vi "waveformGenerator.vi"() -> ()   [LabVIEW 2020]
panel:
  out "Waveform Graph 8":dbl[](graph)
  out "Sawtooth":string
  out "Waveform Graph 7":dbl[](graph)
  out "Square":string
  out "Waveform Graph 6":dbl[](graph)
  out "Camel Sine":string
  out "Waveform Graph 5":dbl[](graph)
  out "Alternating Sine":string
  out "Waveform Graph 4":dbl[](graph)
  out "Pulse Sine":string
  out "Waveform Graph 3":dbl[](graph)
  out "Abs Sine":string
  out "Waveform Graph 2":dbl[](graph)
  out "Half Sine":string
  out "Waveform Graph":dbl[](graph)
  out "Sine":string
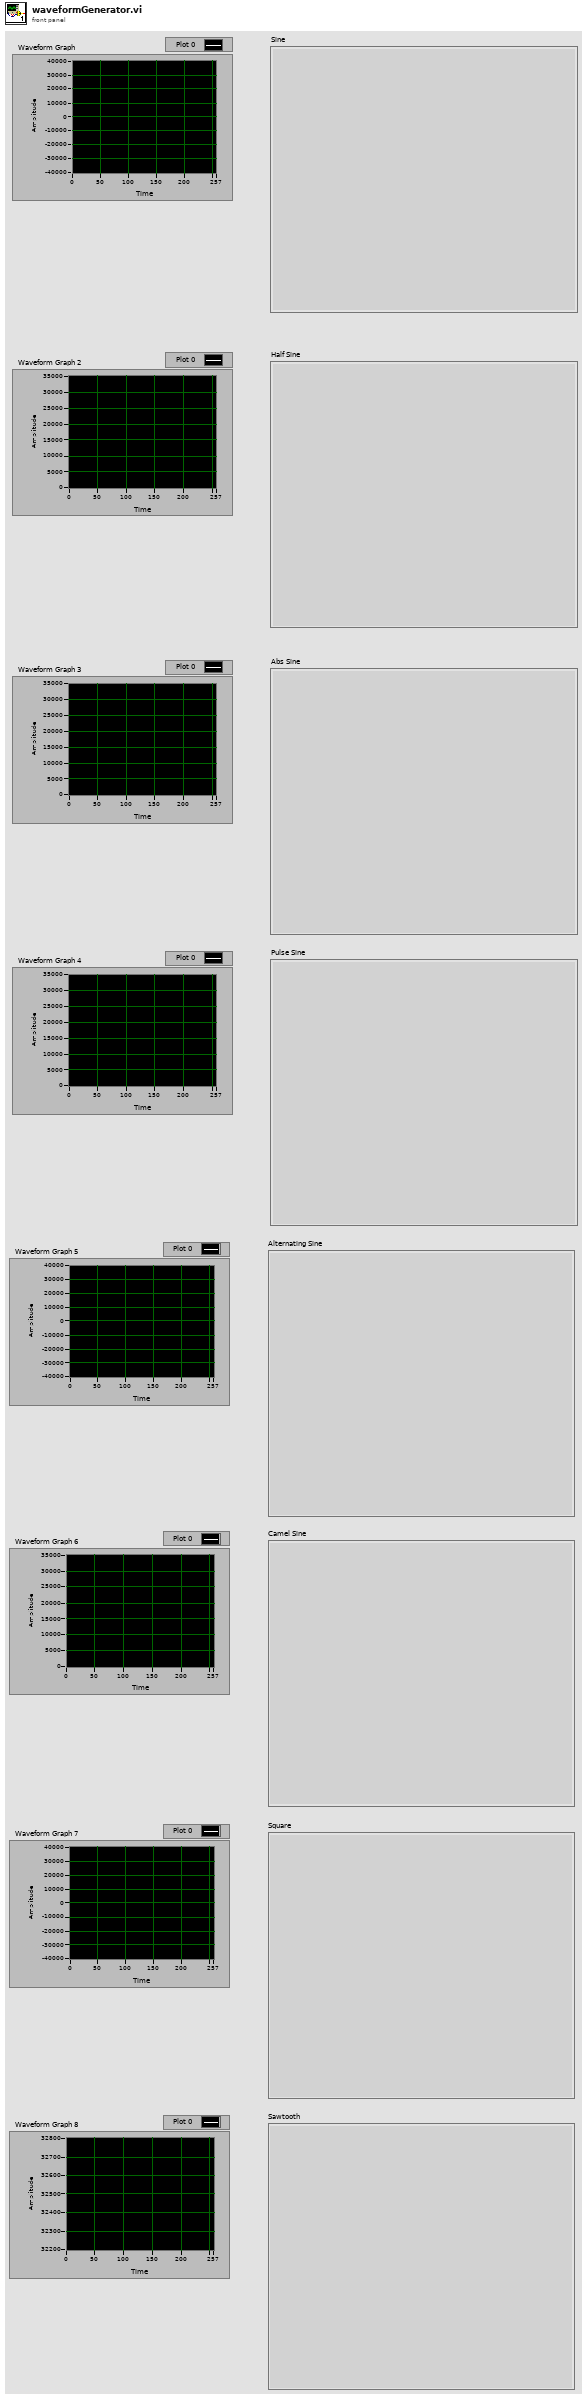
[diagram p1: front panel]
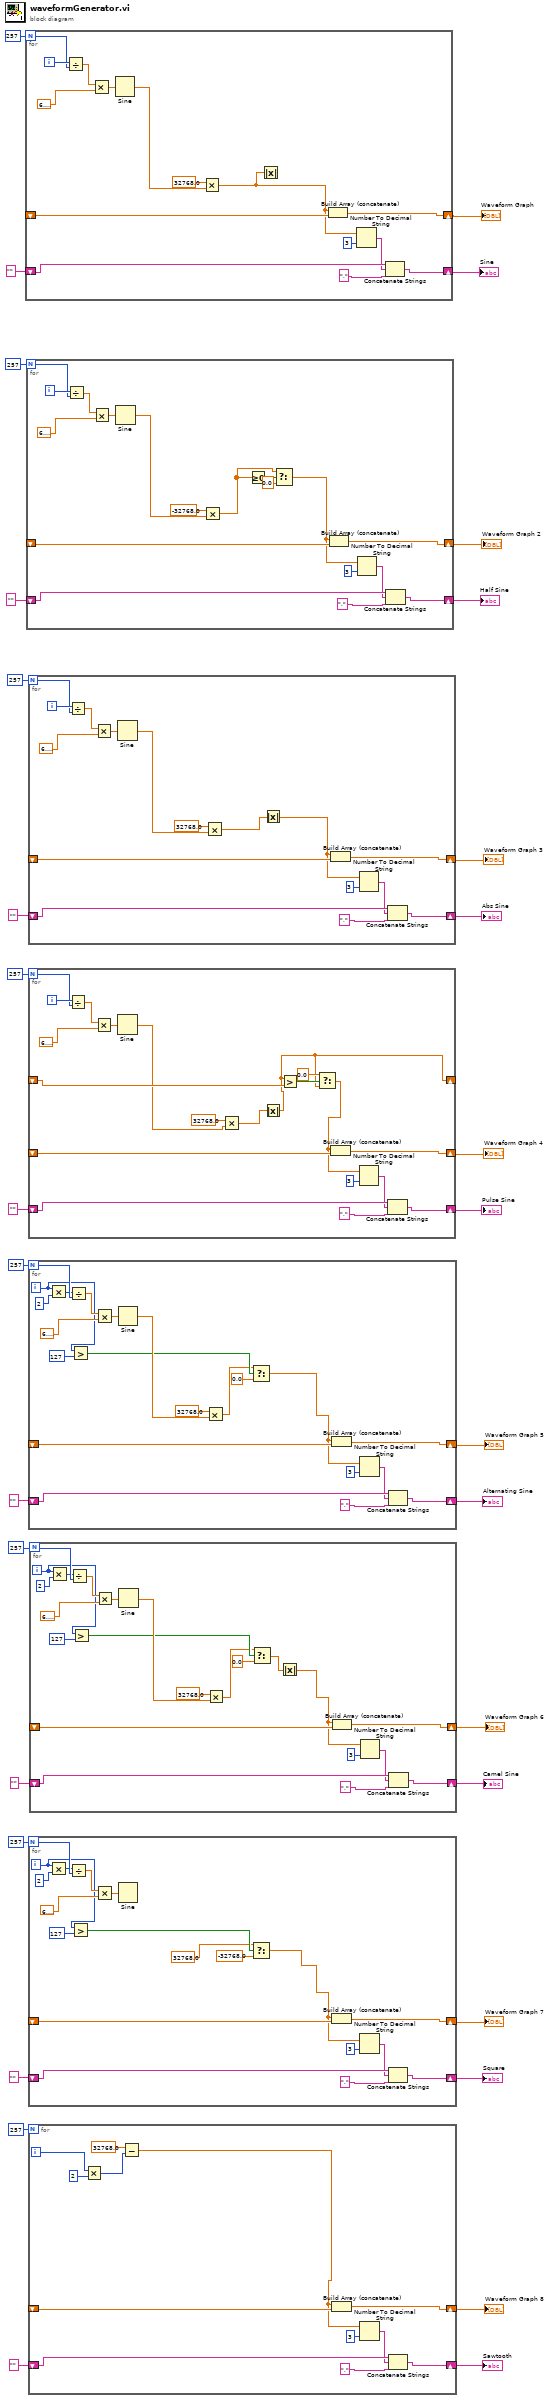
[diagram p0: block diagram]
diagram:
  n1 = for {
    N: 257 -> [w46]
    shift-right: [w39] -> w31
    shift-left: "" ("String") -> [w40]
    shift-right: [w41] -> w29
    shift-left: _ -> [w42]
    i -> [w47]
    n2 = Divide(x=w47, y=w46) -> (x/y=w44:dbl)
    n3 = Multiply(x=w44, y=6.283185307179586) -> (x*y=w43:dbl)
    n4 = Sine(x=w43) -> (sin(x)=w37:dbl)
    n5 = Multiply(x=32768.0, y=w37) -> (x*y=w35:dbl)
    n6 = Absolute Value(x=w35) -> ()  [unwired: 1 out]
    n7 = Build Array (concatenate)(w35, w42) -> (w41:dbl[])
    n8 = Number To Decimal String(number=w35, width (-)=i16 3) -> (decimal integer string=w34:string)
    n9 = Concatenate Strings(w40, w34, "," ("string")) -> (w39:string)
  }
  "Sine" <- w31
  "Waveform Graph" <- w29
  n10 = for {
    N: 257 -> [w64]
    shift-right: [w57] -> w27
    shift-left: "" ("String") -> [w58]
    shift-right: [w59] -> w25
    shift-left: _ -> [w60]
    i -> [w65]
    n11 = Divide(x=w65, y=w64) -> (x/y=w62:dbl)
    n12 = Multiply(x=w62, y=6.283185307179586) -> (x*y=w61:dbl)
    n13 = Sine(x=w61) -> (sin(x)=w55:dbl)
    n14 = Multiply(x=-32768.0, y=w55) -> (x*y=w50:dbl)
    n15 = Greater Or Equal To 0?(x=w50) -> (x >= 0?=w51:bool)
    n16 = Select(t=w50, s=w51, f=0.0) -> (s? t:f=w48:dbl)
    n17 = Build Array (concatenate)(w48, w60) -> (w59:dbl[])
    n18 = Number To Decimal String(number=w48, width (-)=i16 3) -> (decimal integer string=w53:string)
    n19 = Concatenate Strings(w58, w53, "," ("string")) -> (w57:string)
  }
  "Half Sine" <- w27
  "Waveform Graph 2" <- w25
  n20 = for {
    N: 257 -> [w80]
    shift-right: [w73] -> w23
    shift-left: "" ("String") -> [w74]
    shift-right: [w75] -> w21
    shift-left: _ -> [w76]
    i -> [w81]
    n21 = Divide(x=w81, y=w80) -> (x/y=w78:dbl)
    n22 = Multiply(x=w78, y=6.283185307179586) -> (x*y=w77:dbl)
    n23 = Sine(x=w77) -> (sin(x)=w71:dbl)
    n24 = Multiply(x=32768.0, y=w71) -> (x*y=w69:dbl)
    n25 = Absolute Value(x=w69) -> (abs(x)=w66:dbl)
    n26 = Build Array (concatenate)(w66, w76) -> (w75:dbl[])
    n27 = Number To Decimal String(number=w66, width (-)=i16 3) -> (decimal integer string=w68:string)
    n28 = Concatenate Strings(w74, w68, "," ("string")) -> (w73:string)
  }
  "Abs Sine" <- w23
  "Waveform Graph 3" <- w21
  n29 = for {
    N: 257 -> [w100]
    shift-right: [w93] -> w19
    shift-left: "" ("String") -> [w94]
    shift-right: [w95] -> w17
    shift-left: _ -> [w96]
    shift-right: [w82] -> _
    shift-left: _ -> [w87]
    i -> [w101]
    n30 = Divide(x=w101, y=w100) -> (x/y=w98:dbl)
    n31 = Multiply(x=w98, y=6.283185307179586) -> (x*y=w97:dbl)
    n32 = Sine(x=w97) -> (sin(x)=w83:dbl)
    n33 = Multiply(x=32768.0, y=w83) -> (x*y=w90:dbl)
    n34 = Absolute Value(x=w90) -> (abs(x)=w82:dbl)
    n35 = Greater?(x=w82, y=w87) -> (0:w86:bool)
    n36 = Select(t=0.0, s=w86, f=w82) -> (s? t:f=w84:dbl)
    n37 = Build Array (concatenate)(w84, w96) -> (w95:dbl[])
    n38 = Number To Decimal String(number=w84, width (-)=i16 3) -> (decimal integer string=w89:string)
    n39 = Concatenate Strings(w94, w89, "," ("string")) -> (w93:string)
  }
  "Pulse Sine" <- w19
  "Waveform Graph 4" <- w17
  n40 = for {
    N: 257 -> [w122]
    shift-right: [w115] -> w15
    shift-left: "" ("String") -> [w116]
    shift-right: [w117] -> w13
    shift-left: _ -> [w118]
    i -> [w107]
    n41 = Multiply(x=w107, y=2) -> (x*y=w109:i32)
    n42 = Divide(x=w109, y=w122) -> (x/y=w120:dbl)
    n43 = Greater?(x=w107, y=127) -> (0:w105:bool)
    n44 = Multiply(x=w120, y=6.283185307179586) -> (x*y=w119:dbl)
    n45 = Sine(x=w119) -> (sin(x)=w113:dbl)
    n46 = Multiply(x=32768.0, y=w113) -> (x*y=w104:dbl)
    n47 = Select(t=w104, s=w105, f=0.0) -> (s? t:f=w103:dbl)
    n48 = Build Array (concatenate)(w103, w118) -> (w117:dbl[])
    n49 = Number To Decimal String(number=w103, width (-)=i16 3) -> (decimal integer string=w111:string)
    n50 = Concatenate Strings(w116, w111, "," ("string")) -> (w115:string)
  }
  "Alternating Sine" <- w15
  "Waveform Graph 5" <- w13
  n51 = for {
    N: 257 -> [w141]
    shift-right: [w134] -> w7
    shift-left: "" ("String") -> [w135]
    shift-right: [w136] -> w5
    shift-left: _ -> [w137]
    i -> [w128]
    n52 = Multiply(x=w128, y=2) -> (x*y=w130:i32)
    n53 = Divide(x=w130, y=w141) -> (x/y=w139:dbl)
    n54 = Greater?(x=w128, y=127) -> (0:w126:bool)
    n55 = Multiply(x=w139, y=6.283185307179586) -> (x*y=w138:dbl)
    n56 = Sine(x=w138) -> ()  [unwired: 1 out]
    n57 = Select(t=32768.0 ("x"), s=w126, f=-32768.0) -> (s? t:f=w123:dbl)
    n58 = Build Array (concatenate)(w123, w137) -> (w136:dbl[])
    n59 = Number To Decimal String(number=w123, width (-)=i16 3) -> (decimal integer string=w132:string)
    n60 = Concatenate Strings(w135, w132, "," ("string")) -> (w134:string)
  }
  "Square" <- w7
  "Waveform Graph 7" <- w5
  n61 = for {
    N: 257 -> [_]
    shift-right: [w150] -> w3
    shift-left: "" ("String") -> [w151]
    shift-right: [w152] -> w1
    shift-left: _ -> [w153]
    i -> [w145]
    n62 = Multiply(x=w145, y=2) -> (x*y=w144:i32)
    n63 = Subtract(x=32768.0, y=w144) -> (x-y=w142:dbl)
    n64 = Build Array (concatenate)(w142, w153) -> (w152:dbl[])
    n65 = Number To Decimal String(number=w142, width (-)=i16 3) -> (decimal integer string=w148:string)
    n66 = Concatenate Strings(w151, w148, "," ("string")) -> (w150:string)
  }
  "Sawtooth" <- w3
  "Waveform Graph 8" <- w1
  n67 = for {
    N: 257 -> [w175]
    shift-right: [w168] -> w11
    shift-left: "" ("String") -> [w169]
    shift-right: [w170] -> w9
    shift-left: _ -> [w171]
    i -> [w160]
    n68 = Multiply(x=w160, y=2) -> (x*y=w162:i32)
    n69 = Divide(x=w162, y=w175) -> (x/y=w173:dbl)
    n70 = Greater?(x=w160, y=127) -> (0:w158:bool)
    n71 = Multiply(x=w173, y=6.283185307179586) -> (x*y=w172:dbl)
    n72 = Sine(x=w172) -> (sin(x)=w166:dbl)
    n73 = Multiply(x=32768.0, y=w166) -> (x*y=w157:dbl)
    n74 = Select(t=w157, s=w158, f=0.0) -> (s? t:f=w155:dbl)
    n75 = Absolute Value(x=w155) -> (abs(x)=w154:dbl)
    n76 = Build Array (concatenate)(w154, w171) -> (w170:dbl[])
    n77 = Number To Decimal String(number=w154, width (-)=i16 3) -> (decimal integer string=w164:string)
    n78 = Concatenate Strings(w169, w164, "," ("string")) -> (w168:string)
  }
  "Camel Sine" <- w11
  "Waveform Graph 6" <- w9
